vi "USRP Packet Transmitter_BER.vi"() -> ()   [LabVIEW 2013]
uses:
  <vilib>/addons/Modulation/Digital/General/MT Generate PSK System Parameters(M).vi
  <instrlib>/niUSRP/niUSRP Write Tx Data (CDB Cluster).vi
  <vilib>/addons/Modulation/niDMT.lvlib
panel:
  out "Constellation Graph":T1(graph)
  out "Actual Tx Parameters":T2 {"Tx Gain [dB]" format="%#.6p"; "Tx Frequency [Hz]" format="%#.6p"; "Tx IQ Sampling\nRate [s/sec]" format="%#.6p"}
  in  "Tx Parameters":T2={"Tx IQ Sampling\nRate [s/sec]"=200000.0, "Tx Frequency [Hz]"=433920000.0, "Tx Gain [dB]"=0.0, "Tx Antenna"=""} {"Tx Gain [dB]" format="%#.6p"; "Tx Frequency [Hz]" format="%#.6p"; "Tx IQ Sampling\nRate [s/sec]" format="%#.6p"}
  in  "autoscale":bool
  in  "Stop":bool
  in  "USRP IP address":refnum<k15>
  out "Transmitted Signal":cluster{"t0":dbl, "dt":dbl, "Y":dbl[]}(graph)
  in  "Modulation type":string(combo)="QPSK"
  in  "Pulse Shaping\nFilter Parameters":T3={"Alpha"=0.5, "Filter Length"=6, "TX Filter"=enum."Root Raised Cos"} caption="Pulse Shaping Filter" {"Alpha" format="%.2f"}
  out "Symbol Rate [symbols/sec]":dbl=50000.0 format="%#.6p"
  in  "Message Text":string="Two roads diverged in a yellow wood,\nAnd sorry I could not travel both\nAnd be one traveler, long I stood\nAnd looked down one as far as I could\nTo where it bent in the undergrowth.\n\nThen took the other, as just as fair,\nAnd having perhaps the better claim,\nBecause it was grassy and wanted wear;\nThough as for that the passing there\nHad worn them really about the same.\n\nAnd both that morning equally lay\nIn leaves no step had trodden black.\nOh, I kept the first for another day!\nYet knowing how way leads on to way,\nI doubted if I should ever come back.\n\nI shall be telling this with a sigh\nSomewhere ages and ages hence:\nTwo roads diverged in a wood, and I--\nI took the one less traveled by,\nAnd that has made all the difference.\n"
  in  "[Samples]":i32
  out "error out":errorcluster
  in  "Packet Parameters":T4={"Guard Bits "=30, "Sync Bits"=20, "Message Bits"=128}
  in  "Packet Pad [samples]":i32=200
  in  "16-PSK System Parameters":T5={"Samples per Symbol"=8, "symbol map"=[], "Differential PSK"=enum."disable", "PSK type"=0} {"PSK type" items=["normal", "shifted", "offset"]; "symbol map" format="%.3f"}
  in  "8-PSK System Parameters":T5={"Samples per Symbol"=8, "symbol map"=[], "Differential PSK"=enum."disable", "PSK type"=0} {"PSK type" items=["normal", "shifted", "offset"]; "symbol map" format="%.3f"}
  in  "QPSK System Parameters":T5={"Samples per Symbol"=8, "symbol map"=[], "Differential PSK"=enum."disable", "PSK type"=0} {"PSK type" items=["normal", "shifted", "offset"]; "symbol map" format="%.3f"}
  in  "BPSK System Parameters":T5={"Samples per Symbol"=8, "symbol map"=[], "Differential PSK"=enum."disable", "PSK type"=0} {"PSK type" items=["normal", "shifted", "offset"]; "symbol map" format="%.3f"}
  in  "Queue Length":i32=10
  out "Number of Packets in Message":i32=46
  in  "PN sequence order\n for Sync Bits":i32=31 caption="PN sequence order (9)"
  in  "Message Type":bool=TRUE
  # "Pad\nData"
  # "Guard\nBand"
  # "Sync\nSeq"
  # "Packet\nNumber"
  # "Data"
  # "Cyclic Pad"
  # "Guard\nBand"
  # "Sync\nSeq"
  # "Packet\nNumber"
  # "Data"
  # "Packet Transmitter"
  # "Custom Text"
  # "PN Sequence"
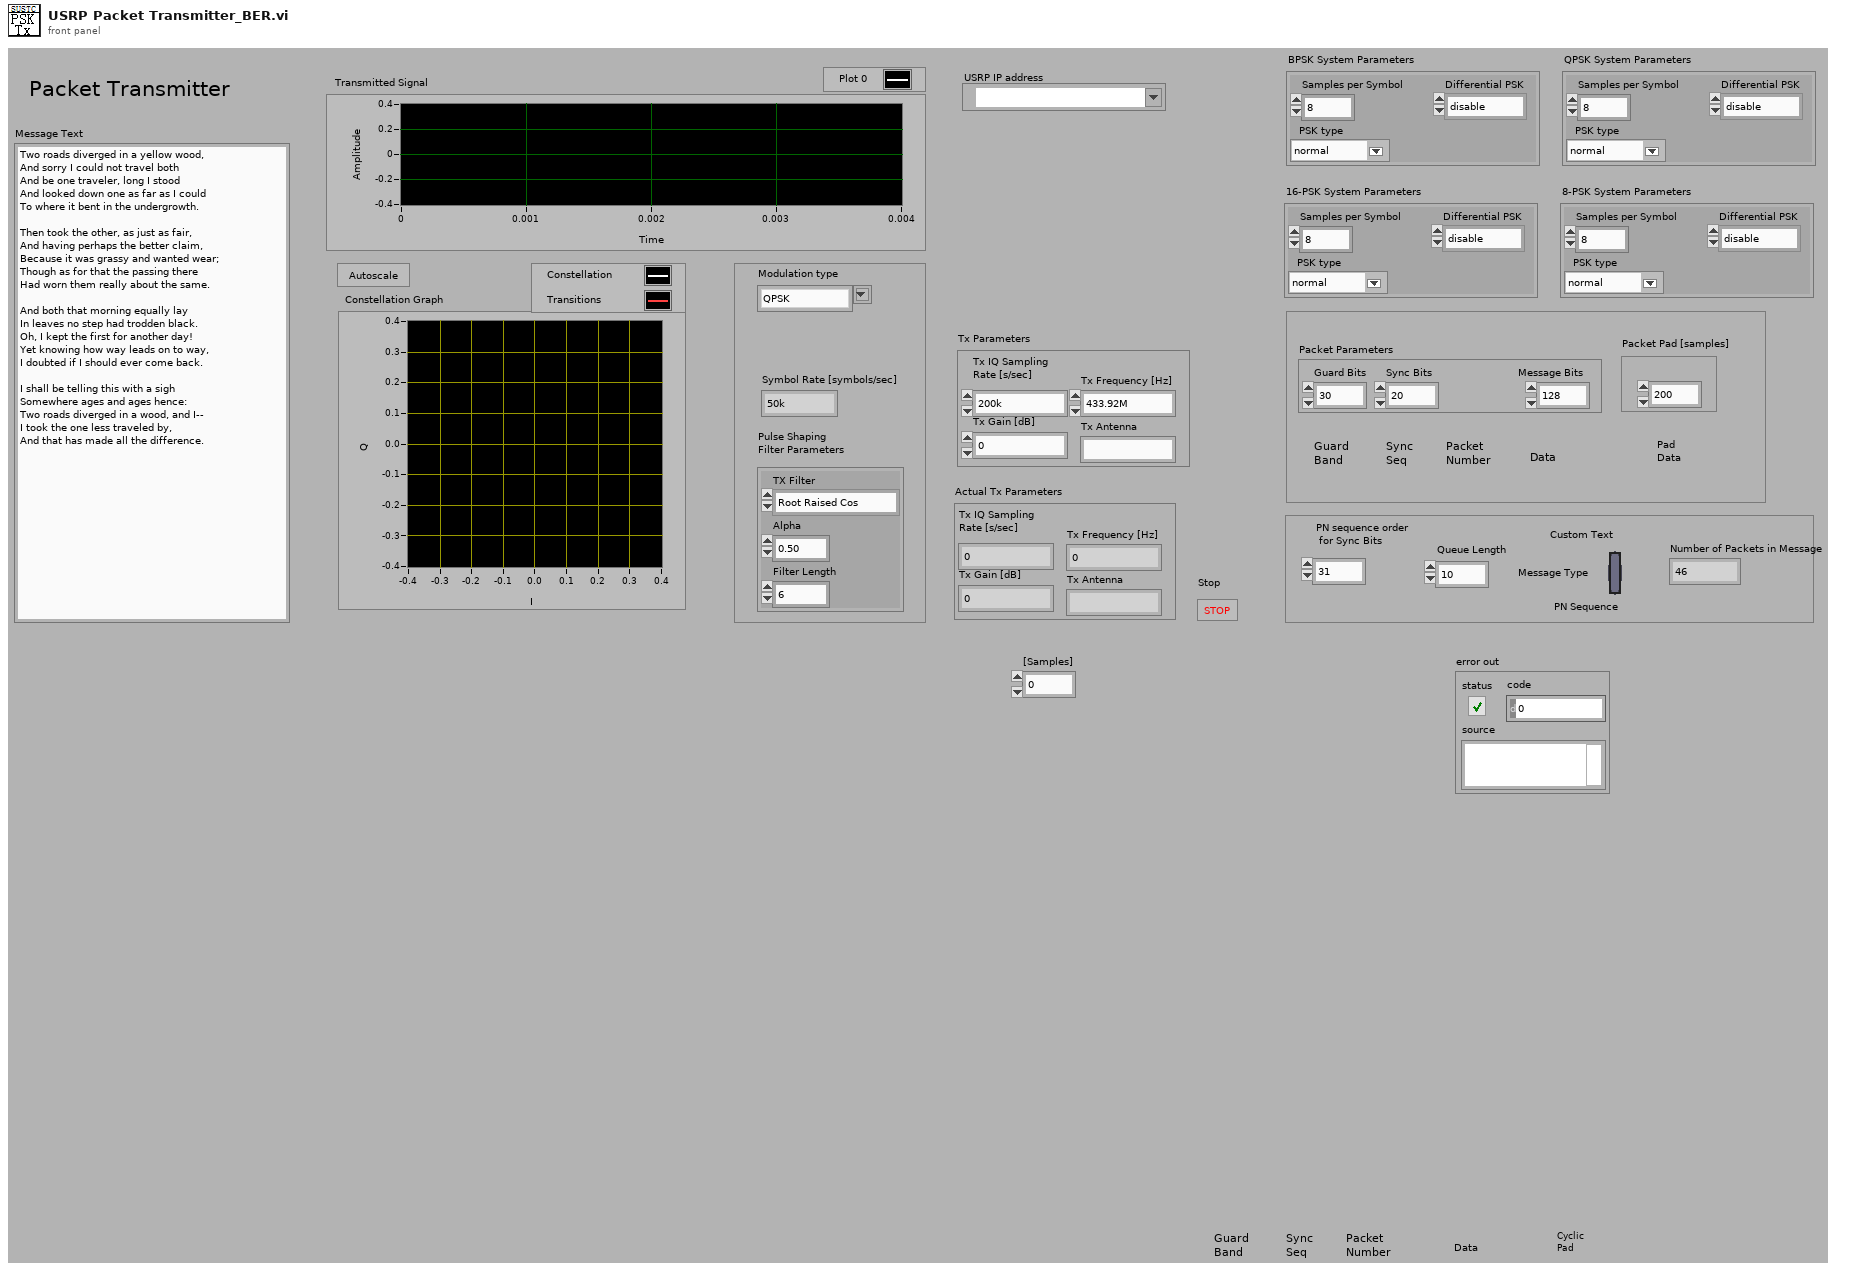
[diagram p1: front panel]
types:
  T1 = cluster{"Decimated Array":dbl[], "Decimated Array":dbl[]}[]
  T2 = cluster{"Tx IQ Sampling\nRate [s/sec]":dbl, "Tx Frequency [Hz]":dbl, "Tx Gain [dB]":dbl, "Tx Antenna":string}
  T3 = cluster{"Alpha":dbl, "Filter Length":i32, "TX Filter":enum16{"none", "Raised Cosine", "Root Raised Cos", "Gaussian"}}
  T4 = cluster{"Guard Bits ":i32, "Sync Bits":i32, "Message Bits":i32}
  T5 = cluster{"Samples per Symbol":i32, "symbol map":cdb[], "Differential PSK":enum16{"disable", "enable"}, "PSK type":u16}
  T6 = cluster{"samples per symbol (16)":i32, "symbol map":cdb[], "differential PSK":enum16{"disable", "enable"}, "PSK type":u16}
  T7 = cluster{"Packet Format":cluster{"t0":dbl, "dt":dbl, "Y":cdb[]}, i32}
  T8 = cluster{"output complex waveform":cluster{"t0":dbl, "dt":dbl, "Y":cdb[]}, i32}
  T9 = cluster{"constellation":dbl[], "oversampled data":dbl[]}[]
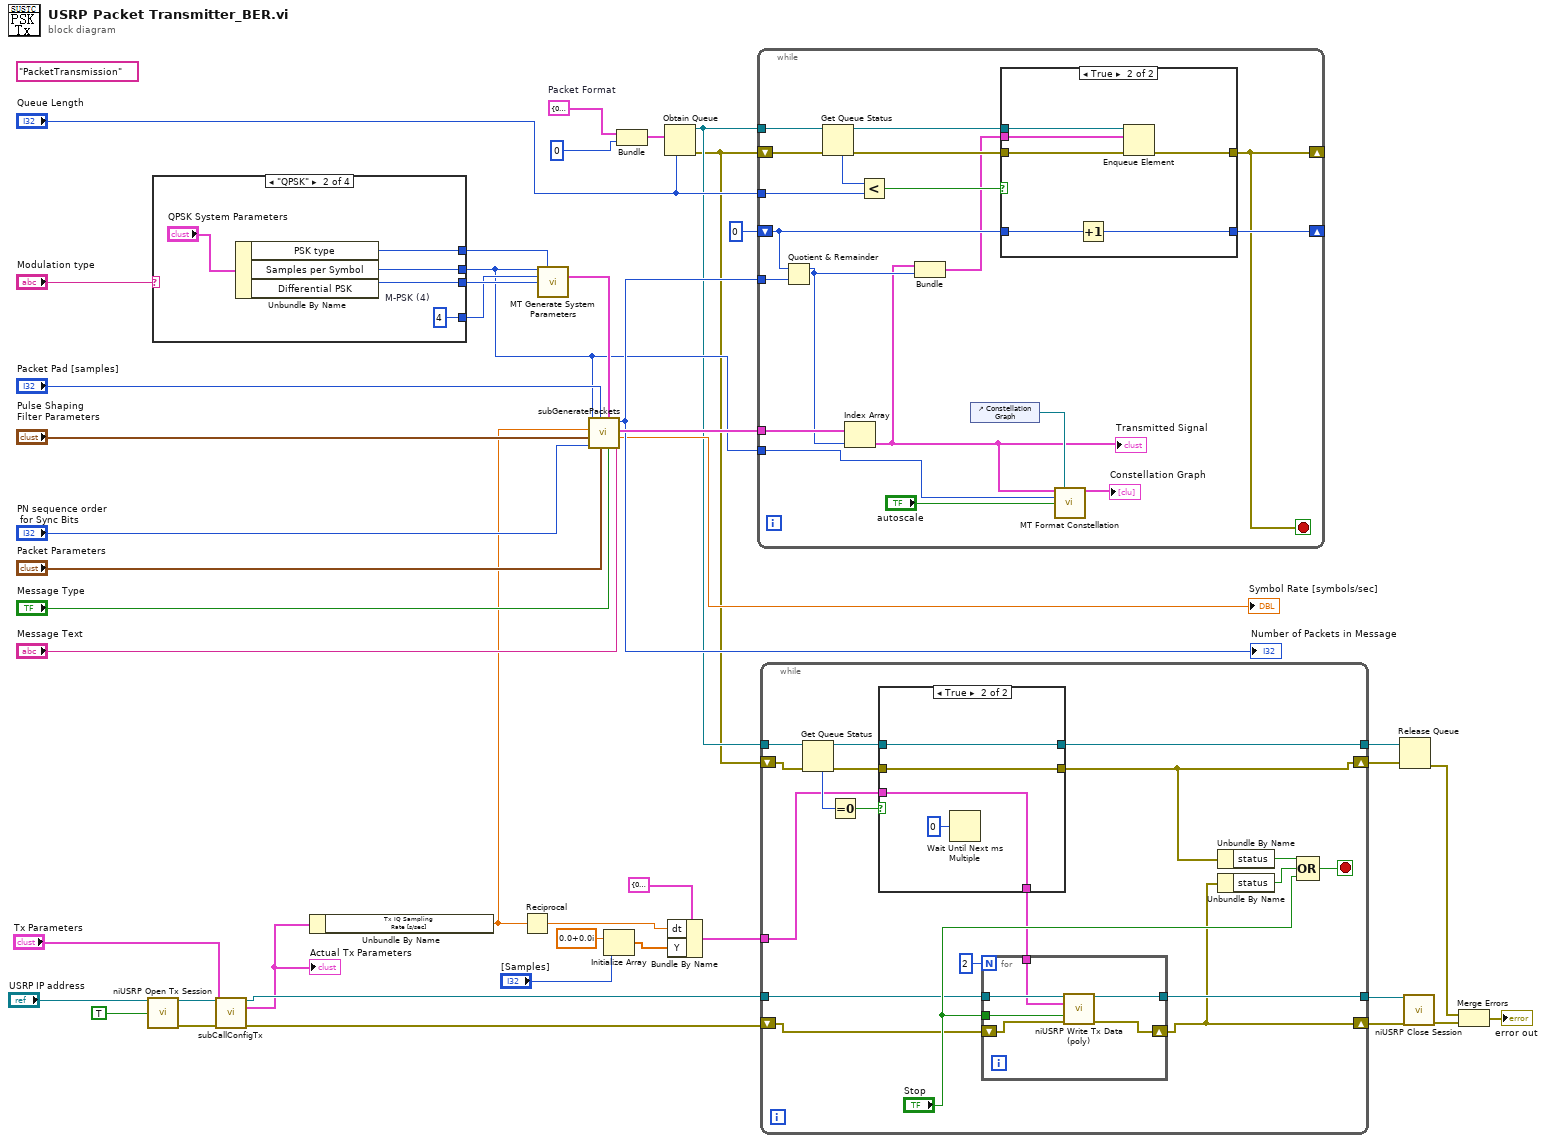
[diagram p0: block diagram]
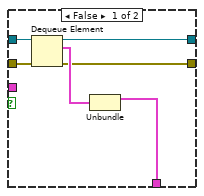
[diagram p2: hidden frame]
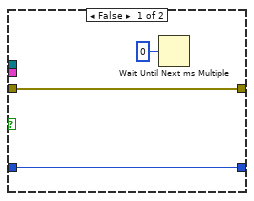
[diagram p3: hidden frame]
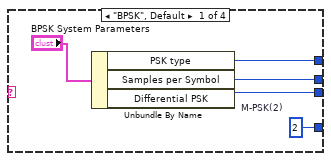
[diagram p4: hidden frame]
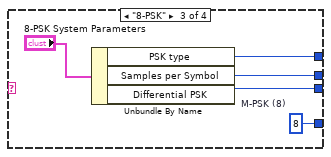
[diagram p5: hidden frame]
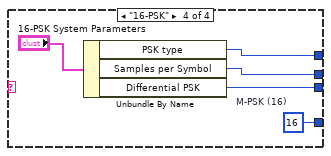
[diagram p6: hidden frame]
diagram:
  (unwired) "PacketTransmission" ("name (unnamed)")
  w15 = cluster{"t0":dbl, "dt":dbl, "Y":cdb[]} {"t0"=0.0, "dt"=0.0, "Y"=[]}  # Packet Format
  n1 = call <instrlib>:"niUSRP Open Tx Session.vi"("device names"="USRP IP address", "reset"=TRUE) -> ("session handle out"=w19:refnum<k15>, "error out"=w18:errorcluster)  [unwired: 12 in]
  n2 = case shown="\"QPSK\"" "Modulation type" {
    tunnel: [w46 w50 w58 w64] -> w30
    tunnel: [w47 w52 w57 w63] -> w44
    tunnel: [w49 w54 w56 w62] -> w39
    tunnel: [w48 w53 w59 w61] -> w34
    frame "BPSK", Default {
      w49 = 2  # M-PSK(2)
      n3 = Unbundle By Name("BPSK System Parameters") -> ("PSK type"=w48:u16, "Samples per Symbol"=w46:i32, "Differential PSK"=w47:enum16{"disable", "enable"})
    }
    frame "QPSK" {
      w54 = 4  # M-PSK (4)
      n4 = Unbundle By Name("QPSK System Parameters") -> ("PSK type"=w53:u16, "Samples per Symbol"=w50:i32, "Differential PSK"=w52:enum16{"disable", "enable"})
    }
    frame "8-PSK" {
      w56 = 8  # M-PSK (8)
      n5 = Unbundle By Name("8-PSK System Parameters") -> ("PSK type"=w59:u16, "Samples per Symbol"=w58:i32, "Differential PSK"=w57:enum16{"disable", "enable"})
    }
    frame "16-PSK" {
      w62 = 16  # M-PSK (16)
      n6 = Unbundle By Name("16-PSK System Parameters") -> ("PSK type"=w61:u16, "Samples per Symbol"=w64:i32, "Differential PSK"=w63:enum16{"disable", "enable"})
    }
  }
  n7 = call "subCallConfigTx.vi"("session handle"=w19, "Tx Parameters"="Tx Parameters", "error in"=w18) -> ("session handle out"=w17:refnum<k15>, "Actual Tx Parameters"=w2:T2, "error out"=w11:errorcluster)  [unwired: 10 in]
  "Actual Tx Parameters" <- w2
  n8 = Unbundle By Name(w2) -> ("Tx IQ Sampling\nRate [s/sec]"=w4:dbl)
  n9 = Reciprocal(x=w4) -> (1/x=w12:dbl)
  n10 = call-poly <vilib>:"MT Generate System Parameters.vi"("samples per symbol (16)"=w30, "PSK type"=w34, "M-PSK (4)"=w39, "differential PSK"=w44) -> ("PSK system parameters"=w35:T6)  [unwired: 9 in, 2 out]
  n11 = call "subGeneratePackets.vi"("Message Text"="Message Text", "Message Type"="Message Type", "PSK system parameters"=w35, "Packet Parameters"="Packet Parameters", "Packet Pad \n[samples]"="Packet Pad [samples]", "PN sequence order\nfor Sync Bits"="PN sequence order\n for Sync Bits", "Pulse Shaping Filter Parameters"="Pulse Shaping\nFilter Parameters", "Tx IQ Sampling\nRate [s/sec]"=w4, "Samples per Symbol"=w30) -> ("Symbol Rate"=→"Symbol Rate [symbols/sec]":dbl, "Packets"=w41:cluster{"t0":dbl, "dt":dbl, "Y":cdb[]}[], "Number of Packets"=w38:i32)
  "Number of Packets in Message" <- w38
  n12 = Initialize Array(csg 0.0+0.0i ("element"), "[Samples]") -> (w13:csg[])
  n13 = Bundle("Packet Format"=w15, 0) -> (w16:T7)  [unwired: 1 in]
  n14 = Obtain Queue(max queue size (-1, unlimited)="Queue Length", element data type=w16) -> (queue out=w25:refnum<queue>, error out=w7:errorcluster)  [unwired: 3 in, 1 out]
  n15 = Bundle By Name "Bundle By Name"(cluster=cluster{"dt":dbl, "t0":dbl, "Y":csg[]} {"dt"=0.0, "t0"=0.0, "Y"=[0.0+0.0i]}, "dt"=w12, "Y"=w13) -> (w5:cluster{"dt":dbl, "t0":dbl, "Y":csg[]})
  n16 = while {
    tunnel: w25 -> [w83]
    shift-right: [w77] -> _
    shift-left: 0 -> [w73]
    tunnel: w41 -> [w74]
    tunnel: "Queue Length" -> [w76]
    tunnel: w38 -> [w75]
    shift-right: [w72] -> _
    shift-left: w7 -> [w78]
    tunnel: w30 -> [w68]
    stop <- w72 stop-if-true
    n17 = Quotient & Remainder(x=w73, y=w75) -> (x-y*floor(x/y)=w69:i32)  [unwired: 1 out]
    n18 = Get Queue Status(queue=w83, error in (no error)=w78) -> (queue out=w82:refnum<queue>, error out=w79:errorcluster, # elements in queue=w81:i32)  [unwired: 1 in, 5 out]
    n19 = Index Array(array=w74, index=w69) -> (element=w65:cluster{"t0":dbl, "dt":dbl, "Y":cdb[]})
    "Transmitted Signal" <- w65
    n20 = Less?(x=w81, y=w76) -> (x < y?=w80:bool)
    n21 = Bundle("output complex waveform"=w65, w69) -> (w70:T8)  [unwired: 1 in]
    n22 = control-ref of="Constellation Graph"() -> (w67:refnum<vi>)
    n23 = case shown="True" w80 {
      tunnel: w79 -> [w85 w92]
      tunnel: w82 -> [_ w91]
      tunnel: [w85 w90] -> w72
      tunnel: w70 -> [_ w89]
      tunnel: w73 -> [w86 w88]
      tunnel: [w86 w87] -> w77
      frame False {
        n24 = Wait Until Next ms Multiple(millisecond multiple=u32 0) -> ()  [unwired: 1 out]
      }
      frame True {
        n25 = Increment(x=w88) -> (x+1=w87:i32)
        n26 = Enqueue Element(queue=w91, element=w89, error in (no error)=w92) -> (error out=w90:errorcluster)  [unwired: 1 in, 2 out]
      }
    }
    n27 = call <vilib>:"MT Format Constellation.vi"("waveform"=w65, "constellation reference"=w67, "samples per symbol"=w68, "autoscale"="autoscale") -> ("constellation graph"=→"Constellation Graph":T9)  [unwired: 10 in, 1 out]
  }
  n28 = while {
    tunnel: w25 -> [w109]
    tunnel: [w105] -> w9
    tunnel: w17 -> [w102]
    shift-right: [w99] -> w10
    shift-left: w11 -> [w100]
    shift-right: [w93] -> w8
    shift-left: w7 -> [w98]
    tunnel: w5 -> [w97]
    tunnel: [w95] -> w1
    stop <- w104 stop-if-true
    n29 = Get Queue Status(queue=w109, error in (no error)=w98) -> (queue out=w111:refnum<queue>, error out=w110:errorcluster, # elements in queue=w107:i32)  [unwired: 1 in, 5 out]
    n30 = Equal To 0?(x=w107) -> (x = 0?=w108:bool)
    n31 = case shown="True" w108 {
      tunnel: w111 -> [w122 w127]
      tunnel: w110 -> [w118 w126]
      tunnel: w97 -> [_ w125]
      tunnel: [w121 w127] -> w95
      tunnel: [w120 w126] -> w93
      tunnel: [w119 w125] -> w94
      frame False {
        n32 = Dequeue Element(queue=w122, error in (no error)=w118) -> (queue out=w121:refnum<queue>, element=w123:T7, error out=w120:errorcluster)  [unwired: 1 in, 1 out]
        n33 = Unbundle(w123) -> ("Packet Format"=w119:cluster{"t0":dbl, "dt":dbl, "Y":cdb[]})  [unwired: 1 out]
      }
      frame True {
        n34 = Wait Until Next ms Multiple(millisecond multiple=u32 0) -> ()  [unwired: 1 out]
      }
    }
    n35 = for {
      N: 2 -> [_]
      tunnel: [w117] -> w105
      tunnel: "Stop" -> [w116]
      tunnel: w102 -> [w115]
      shift-right: [w113] -> w99
      shift-left: w100 -> [w114]
      tunnel: w94 -> [w112]
      n36 = call-poly <instrlib>:"niUSRP Write Tx Data (poly).vi"("session handle"=w115, "data"=w112, "end of data?"=w116, "error in (no error)"=w114) -> ("session handle out"=w117:refnum<k15>, "error out"=w113:errorcluster)  [unwired: 10 in]
    }
    n37 = Unbundle By Name(w93) -> ("status"=w101:bool)
    n38 = Unbundle By Name(w99) -> ("status"=w96:bool)
    n39 = Compound Arithmetic op=OR(w101, w96, "Stop") -> (w104:bool)
  }
  n40 = Release Queue(queue=w1, error in (no error)=w8) -> (error out=w23:errorcluster)  [unwired: 1 in, 2 out]
  n41 = call <instrlib>:"niUSRP Close Session.vi"("session handle"=w9, "error in (no error)"=w10) -> ("error out"=w24:errorcluster)  [unwired: 13 in]
  n42 = Merge Errors(w23, w24) -> (→"error out":errorcluster)
